vi "USB_DAQ__DS3231_RTC_Test_READ_Date_Time.vi"() -> ()   [LabVIEW 2022 SP3]
doc: "Petrus Prins\n26 July 2026"
uses:
  <vilib>/MakerHub/Toolbox/LMH-Toolbox.lvlib
panel:
  out "Data_Valid":bool
  out "Raw_RTC_Data":u8[](array[numeric]) format="%2x"
  in  "Read Time":bool
  out "DegC":dbl format="%-2_6g"
  out "Temp_Valid":bool
  in  "Device.Addr":u8=104 format="%x"
  in  "Stop":bool
  in  "Read Temp":bool
  # "DS3231"
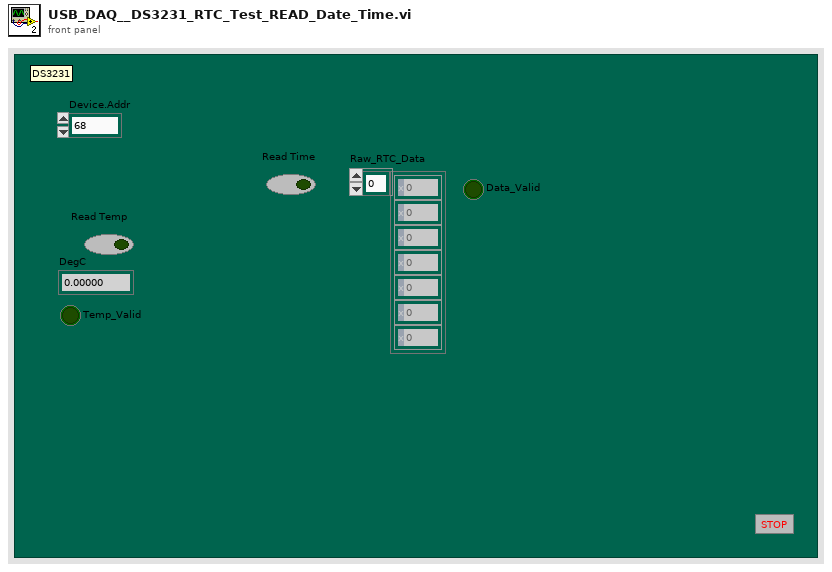
[diagram p1: front panel]
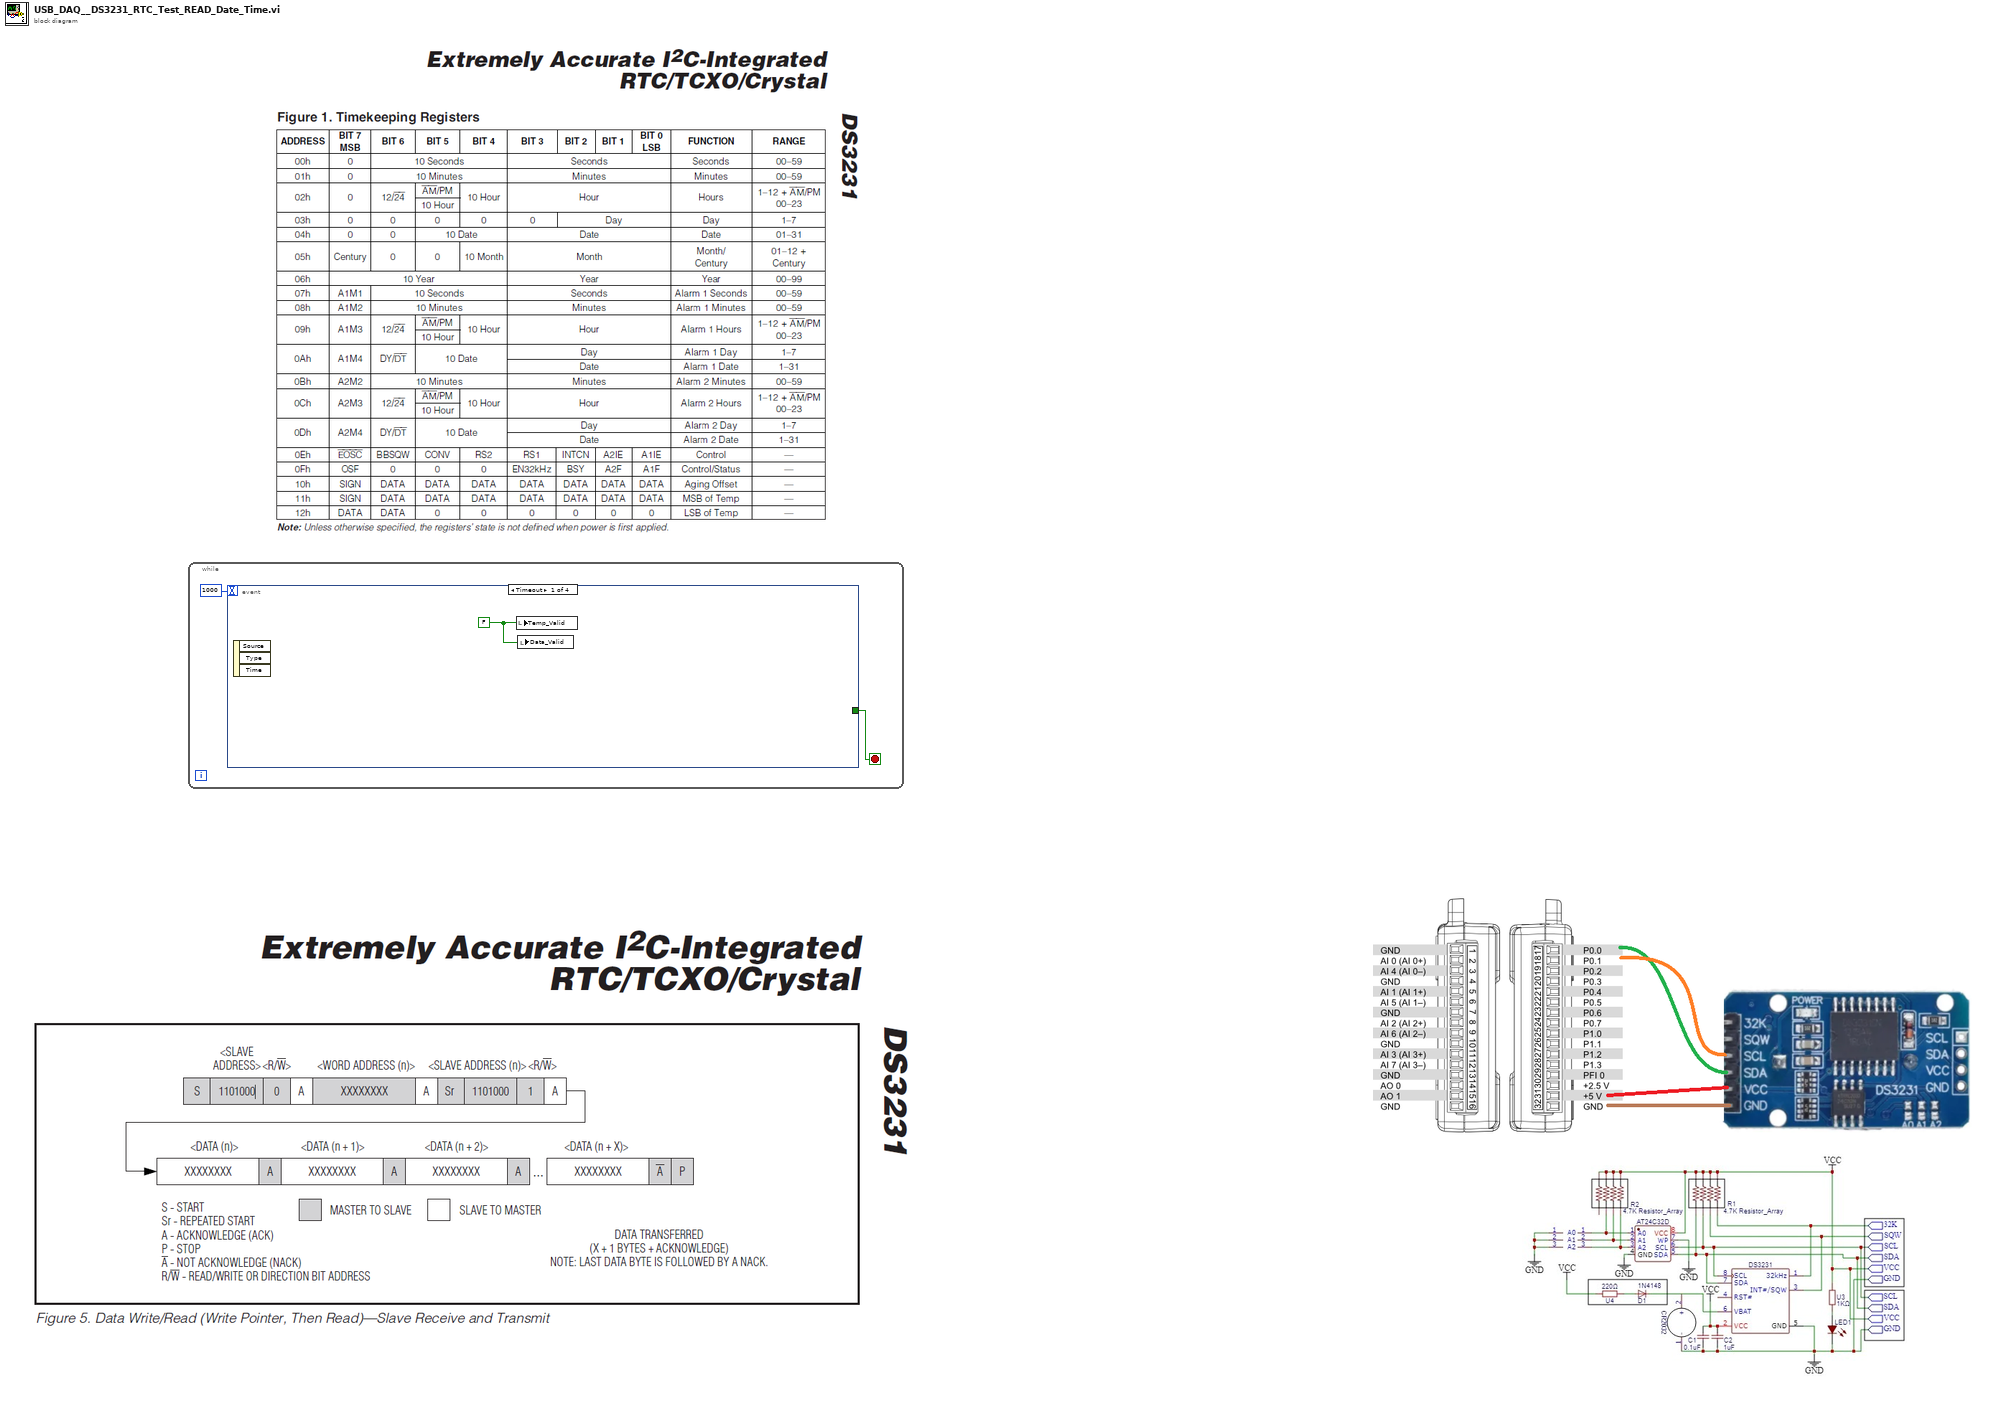
[diagram p0: block diagram]
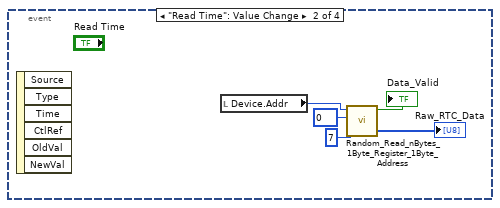
[diagram p2: hidden frame]
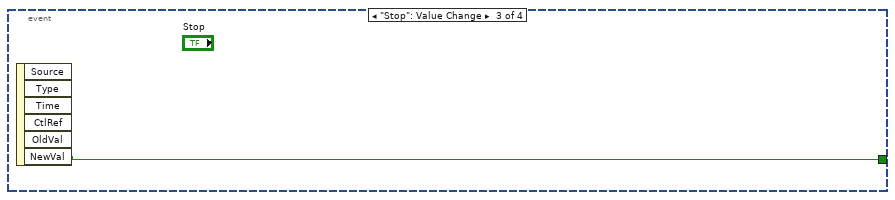
[diagram p3: hidden frame]
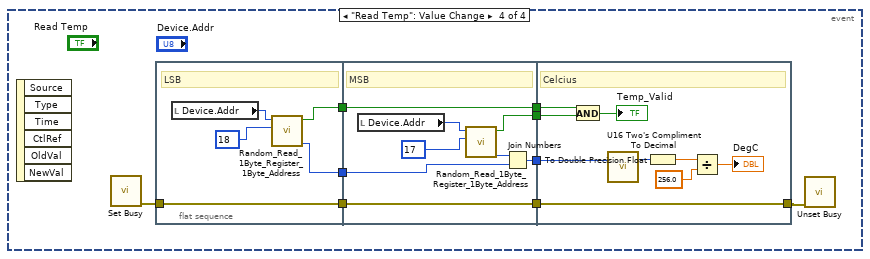
[diagram p4: hidden frame]
diagram:
  n1 = while {
    stop <- w1 stop-if-true
    n2 = event shown="[0] Timeout" {
      selector: _ -> [_ _ _ _]
      dyn-events: _ -> [_ _ _ _]
      timeout: 1000 -> [_ _ _ _]
      tunnel: [_ _ w9 _] -> w1
      event Timeout {
        w3 = FALSE ("Temp_Valid")
        n3 = event-data() -> ()  [unwired: 1 in, 3 out]
        n4 = local write "Temp_Valid"(w3) -> ()
        n5 = local write "Data_Valid"(w3) -> ()
      }
      event "Read Time": Value Change {
        n6 = event-data() -> ()  [unwired: 1 in, 6 out]
        n7 = local read "Device.Addr"() -> (w8:u8)
        n8 = call "Random_Read_nBytes_1Byte_Register_1Byte_Address.vi"("Rx.Byte.Count.In"=7, "Register.Addr"=u8 0, "Device.Addr"=w8) -> ("Rx.Array.Out"=→"Raw_RTC_Data":u8[], "Data_Valid"=→"Data_Valid":bool)  [unwired: 4 in]
      }
      event "Stop": Value Change {
        n9 = event-data() -> ("NewVal"=w9:bool)  [unwired: 1 in, 5 out]
      }
      event "Read Temp": Value Change {
        n10 = event-data() -> ()  [unwired: 1 in, 6 out]
        n11 = call <vilib>:"Set Busy.vi"() -> ("error out"=w13:errorcluster)  [unwired: 10 in, 1 out]
        n12 = flat-sequence {
          tunnel: [w21] -> w18
          tunnel: [w20] -> w15
          tunnel: w13 -> [w19]
          tunnel: [w19] -> w11
          tunnel: w18 -> [w29]
          tunnel: [w29] -> w17
          tunnel: [w28] -> w16
          tunnel: w15 -> [w25]
          tunnel: [w27] -> w14
          tunnel: [w24] -> w12
          tunnel: w11 -> [w24]
          tunnel: w17 -> [w38]
          tunnel: w16 -> [w39]
          tunnel: w14 -> [w33]
          tunnel: [w32] -> w10
          tunnel: w12 -> [w32]
          frame #0 {
            # "LSB"
            n13 = local read "Device.Addr"() -> (w23:u8)
            n14 = call "Random_Read_1Byte_Register_1Byte_Address.vi"("Register.Addr"=u8 18 ("Device.Addr"), "Device.Addr"=w23) -> ("Data.Byte.Read"=w20:u8, "Data_Valid"=w21:bool)  [unwired: 5 in]
          }
          frame #1 {
            # "MSB"
            n15 = local read "Device.Addr"() -> (w31:u8)
            n16 = call "Random_Read_1Byte_Register_1Byte_Address.vi"("Register.Addr"=u8 17 ("Device.Addr"), "Device.Addr"=w31) -> ("Data.Byte.Read"=w26:u8, "Data_Valid"=w28:bool)  [unwired: 5 in]
            n17 = Join Numbers(hi=w26, lo=w25) -> ((hi.lo)=w27:u16)
          }
          frame #2 {
            # "Celcius"
            n18 = And(x=w38, y=w39) -> (x .and. y?=→"Temp_Valid":bool)
            n19 = call <vilib>:"U16 Two's Compliment To Decimal.vi"("Two's Compliment U16"=w33) -> ("Decimal I16"=w37:i16)  [unwired: 2 in]
            n20 = To Double Precision Float(number=w37) -> (double precision float=w36:dbl)
            n21 = Divide(x=w36, y=256.0) -> (x/y=→"DegC":dbl)
          }
        }
        n22 = call <vilib>:"Unset Busy.vi"("error in (no error)"=w10) -> ()  [unwired: 10 in, 1 out]
      }
    }
  }
